vi "Initialise DVRs.vi"(8 "error in (no error)":errorcluster) -> (0 "error out":errorcluster, 3 "Data":T1)   [LabVIEW 2021, in "Blackboard.lvclass"]
uses:
  Blackboard.lvclass
  Data DVR Type.ctl
  Tags Map Type.ctl
  Status Type.ctl
  Data Type.ctl
  Blackboard.lvclass/Blackboard.ctl
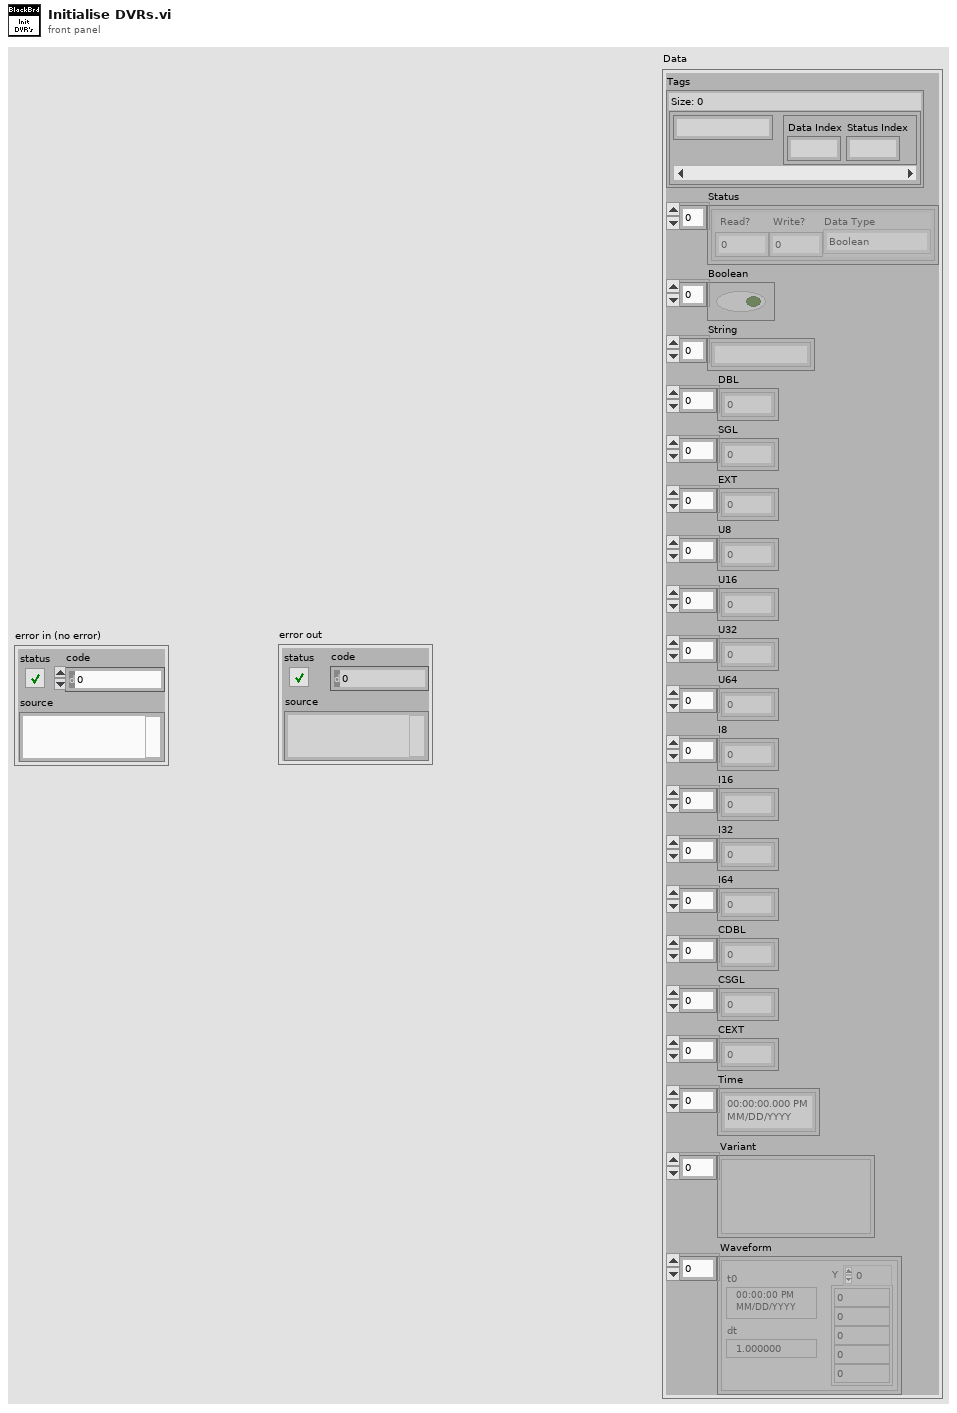
[diagram p1: front panel]
types:
  T1 = typedef "Blackboard.lvclass/Data DVR Type.ctl" = cluster{"Tags":T2, "Status":T3[], "Boolean":bool[], "String":string[], "DBL":dbl[], "SGL":sgl[], "EXT":ext[], "U8":u8[], "U16":u16[], "U32":u32[], "U64":u64[], "I8":i8[], "I16":i16[], "I32":i32[], "I64":i64[], "CDBL":cdb[], "CSGL":csg[], "CEXT":cxt[], "Time":timestamp[], "Variant":variant[], "Waveform":waveform(dbl)[]}
  T2 = typedef "Blackboard.lvclass/Tags Map Type.ctl" = map{string, cluster{"Data Index":i32, "Status Index":i32}}
  T3 = typedef "Blackboard.lvclass/Status Type.ctl" = cluster{"Read?":u32, "Write?":u32, "Data Type":T4}
  T4 = typedef "Blackboard.lvclass/Data Type.ctl" = enum16{"Boolean", "String", "DBL", "SGL", "EXT", "U8", "U16", "U32", "U64", "I8", "I16", "I32", "I64", "CDBL", "CSGL", "CEXT", "Time", "Variant", "Waveform"}
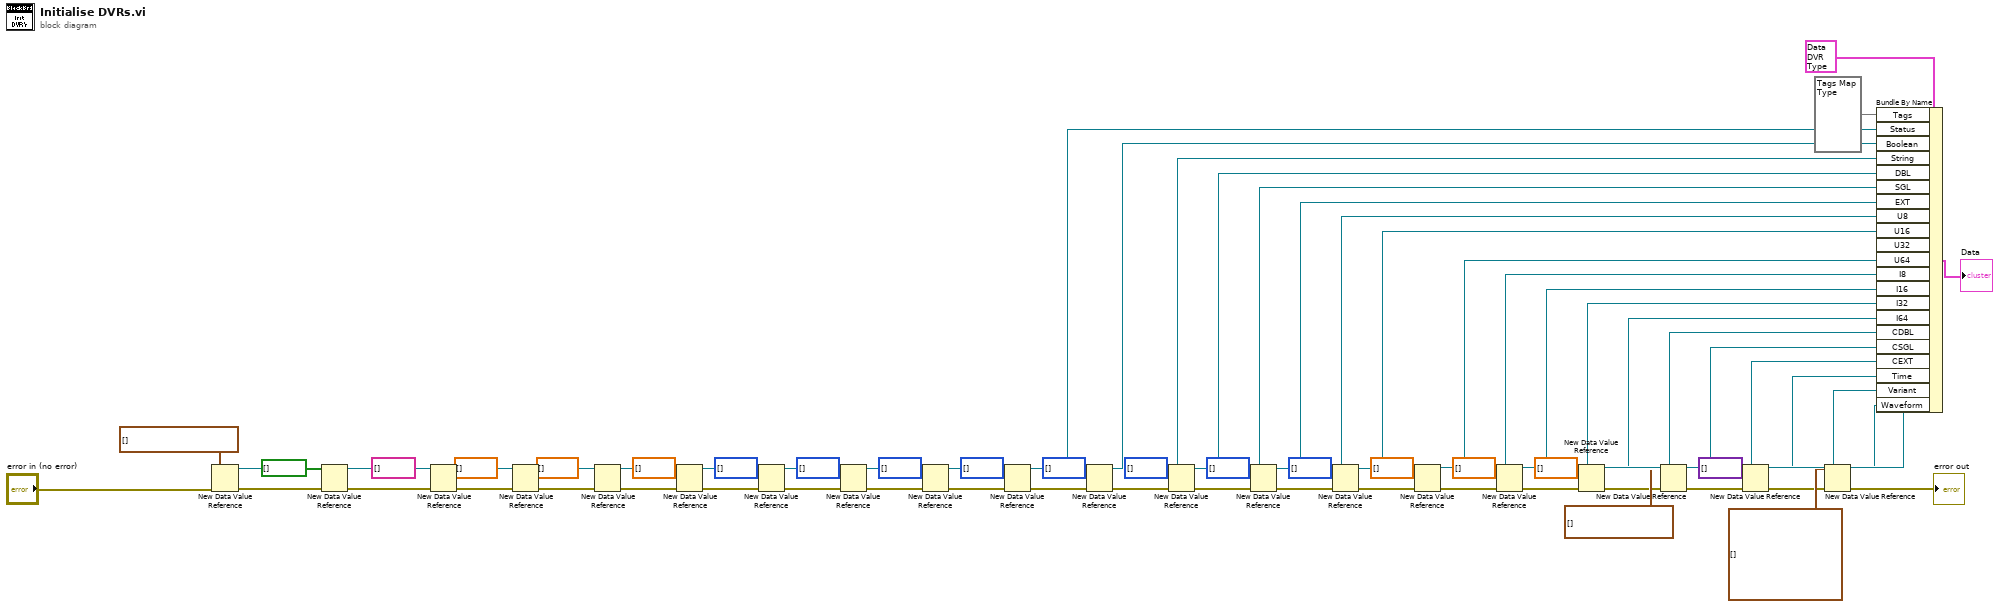
[diagram p0: block diagram]
diagram:
  n1 = New Data Value Reference(data value=T3[] [] ("Array"), error in="error in (no error)") -> (data value reference=w3:refnum<data-value>, error out=w4:errorcluster)
  n2 = New Data Value Reference(data value=bool[] [], error in=w4) -> (data value reference=w61:refnum<data-value>, error out=w59:errorcluster)
  n3 = New Data Value Reference(data value=string[] [], error in=w59) -> (data value reference=w58:refnum<data-value>, error out=w56:errorcluster)
  n4 = New Data Value Reference(data value=dbl[] [], error in=w56) -> (data value reference=w55:refnum<data-value>, error out=w16:errorcluster)
  n5 = New Data Value Reference(data value=sgl[] [], error in=w16) -> (data value reference=w48:refnum<data-value>, error out=w15:errorcluster)
  n6 = New Data Value Reference(data value=ext[] [], error in=w15) -> (data value reference=w47:refnum<data-value>, error out=w14:errorcluster)
  n7 = New Data Value Reference(data value=u8[] [], error in=w14) -> (data value reference=w46:refnum<data-value>, error out=w13:errorcluster)
  n8 = New Data Value Reference(data value=u16[] [], error in=w13) -> (data value reference=w45:refnum<data-value>, error out=w12:errorcluster)
  n9 = New Data Value Reference(data value=u32[] [], error in=w12) -> (data value reference=w44:refnum<data-value>, error out=w11:errorcluster)
  n10 = New Data Value Reference(data value=u64[] [], error in=w11) -> (data value reference=w43:refnum<data-value>, error out=w10:errorcluster)
  n11 = New Data Value Reference(data value=i8[] [], error in=w10) -> (data value reference=w38:refnum<data-value>, error out=w9:errorcluster)
  n12 = New Data Value Reference(data value=i16[] [], error in=w9) -> (data value reference=w37:refnum<data-value>, error out=w8:errorcluster)
  n13 = New Data Value Reference(data value=i32[] [], error in=w8) -> (data value reference=w36:refnum<data-value>, error out=w7:errorcluster)
  n14 = New Data Value Reference(data value=i64[] [], error in=w7) -> (data value reference=w35:refnum<data-value>, error out=w6:errorcluster)
  n15 = New Data Value Reference(data value=cdb[] [], error in=w6) -> (data value reference=w31:refnum<data-value>, error out=w17:errorcluster)
  n16 = New Data Value Reference(data value=csg[] [], error in=w17) -> (data value reference=w30:refnum<data-value>, error out=w18:errorcluster)
  n17 = New Data Value Reference(data value=cxt[] [], error in=w18) -> (data value reference=w29:refnum<data-value>, error out=w19:errorcluster)
  n18 = New Data Value Reference(data value=timestamp[] [], error in=w19) -> (data value reference=w25:refnum<data-value>, error out=w20:errorcluster)
  n19 = New Data Value Reference(data value=variant[] [], error in=w20) -> (data value reference=w24:refnum<data-value>, error out=w21:errorcluster)
  n20 = New Data Value Reference(data value=waveform(dbl)[] [], error in=w21) -> (data value reference=w23:refnum<data-value>, error out=→"error out":errorcluster)
  n21 = Bundle By Name(cluster=T1 {"Tags"={}, "Status"=[], "Boolean"=[], "String"=[], "DBL"=[], "SGL"=[], "EXT"=[], "U8"=[], "U16"=[], "U32"=[], "U64"=[], "I8"=[], "I16"=[], "I32"=[], "I64"=[], "CDBL"=[], "CSGL"=[], "CEXT"=[], "Time"=[], "Variant"=[], "Waveform"=[]} ("Data"), "Tags"=T2 {}, "Status"=w3, "Boolean"=w61, "String"=w58, "DBL"=w55, "SGL"=w48, "EXT"=w47, "U8"=w46, "U16"=w45, "U32"=w44, "U64"=w43, "I8"=w38, "I16"=w37, "I32"=w36, "I64"=w35, "CDBL"=w31, "CSGL"=w30, "CEXT"=w29, "Time"=w25, "Variant"=w24, "Waveform"=w23) -> (→"Data":T1)
